vi "Write Control to write_.vi"(8 "error in (no error)":errorcluster, 10 "Control to write?":bool, 11 "Modbus in":refnum<class "Modbus.lvclass">) -> (0 "error out":errorcluster, 3 "Modbus out":refnum<class "Modbus.lvclass">)   [LabVIEW 2020, in "Modbus.lvlib" / "Modbus.lvclass"]
uses:
  Modbus.lvclass
  Modbus.lvclass/Modbus.ctl
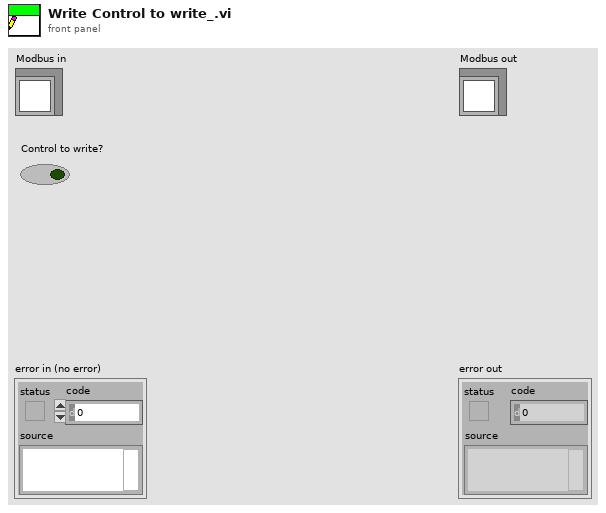
[diagram p1: front panel]
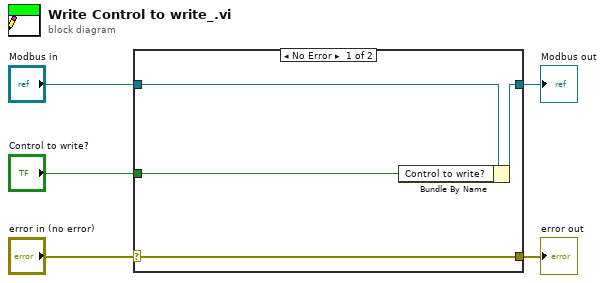
[diagram p0: block diagram]
diagram:
  n1 = case shown="No Error" "error in (no error)" {
    selector: "error in (no error)" -> [w9 w10]
    tunnel: [w9 w10] -> w4
    tunnel: [w7 w11] -> w2
    tunnel: "Modbus in" -> [w8 w11]
    tunnel: "Control to write?" -> [w6 _]
    frame No Error {
      n2 = Bundle By Name(cluster=w8, "Control to write?"=w6) -> (w7:refnum<class "Modbus.lvclass">)
    }
    frame Error {
    }
  }
  "error out" <- w4
  "Modbus out" <- w2
